vi "Release Buffers.vi"(8 "error in (no error)":errorcluster, 11 "Historian Module in":refnum<class "Historian Module.lvclass">) -> (0 "error out":errorcluster, 3 "Historian Module out":refnum<class "Historian Module.lvclass">)   [LabVIEW 2020, in "VolatusHistorian.lvlib" / "Historian Module.lvclass"]
uses:
  Historian Module.lvclass
  Historian Module.lvclass/Historian Module.ctl
  Group Buffer DBL/Group Buffer DBL.lvclass
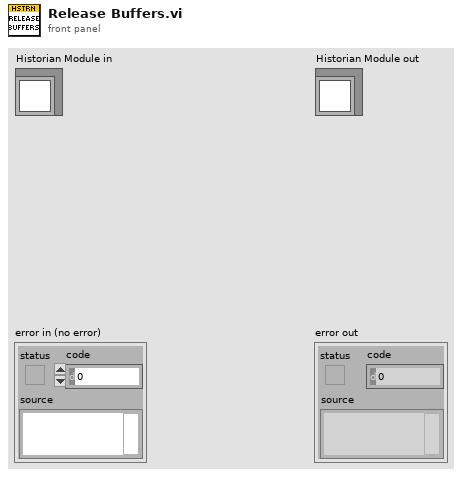
[diagram p1: front panel]
types:
  T1 = map{string, refnum<class "Group Buffer DBL.lvclass">}
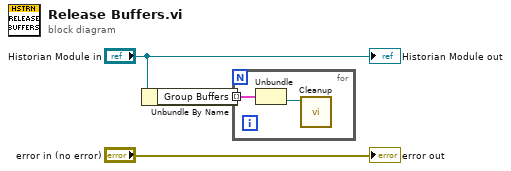
[diagram p0: block diagram]
diagram:
  n1 = Unbundle By Name("Historian Module in") -> ("Group Buffers"=w1:T1)
  n2 = for {
    tunnel: w1 -> [w5] mode=indexing
    n3 = Unbundle(w5) -> ("Buffer"=w4:refnum<class "Group Buffer DBL.lvclass">)  [unwired: 1 out]
    n4 = call "Cleanup.vi"("Group Buffer DBL in"=w4) -> ()  [unwired: 10 in, 1 out]
  }
  "error out" <- "error in (no error)"
  "Historian Module out" <- "Historian Module in"
